vi "TestTriggerTimestamp.vi"() -> ()   [LabVIEW 2014]
uses:
  <instrlib>/niSync/niSync.llb/niSync Initialize (IVI).vi
  <instrlib>/niSync/niSync.llb/niSync Set Time Reference (GPS).vi
  <instrlib>/niSync/niSync.llb/niSync Create Clock (Frequency).vi
  <instrlib>/niSync/niSync.llb/niSync Read Trigger Time Stamp (Single).vi
panel:
  out "Final error":errorcluster
  out "Connection Error":errorcluster
  in  "source terminal":string(combo)="PXI_Trig2"
  out "Stop":bool
  out "Pause Error":errorcluster
  out "Play Error":errorcluster
  in  "Trigger Terminal":tag="/PXI1Slot7/PFI1"
  in  "Reference Clock":refnum<k15>="PXI1Slot7"
  out "time stamp out":timestamp
  out "Read Error":errorcluster
  in  "Pause Button":bool
  in  "Play Button":bool
  in  "Stop Button":bool
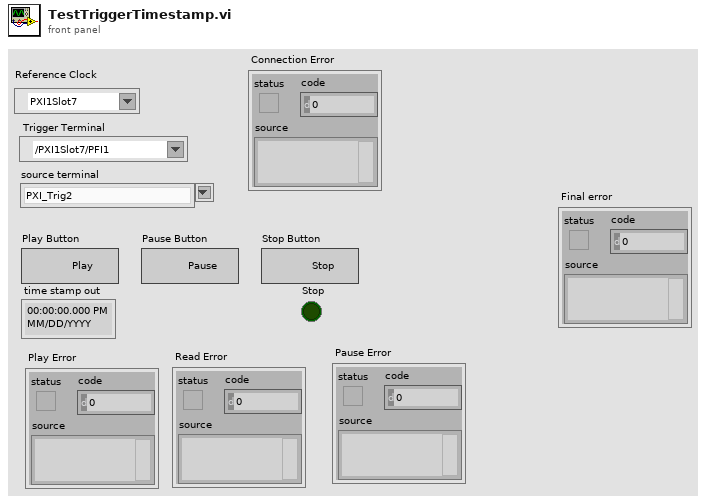
[diagram p1: front panel]
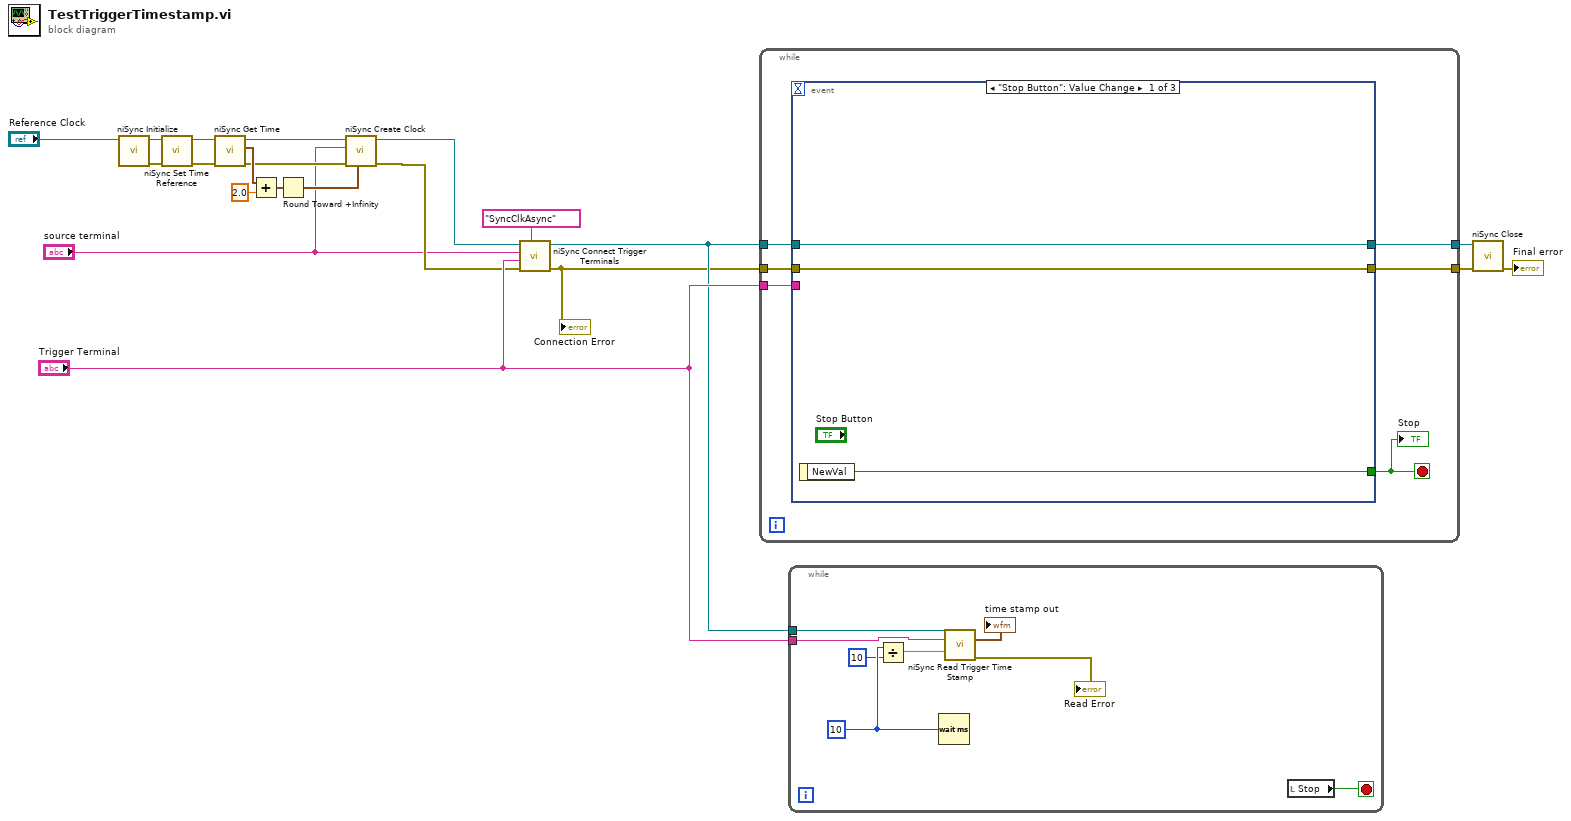
[diagram p0: block diagram]
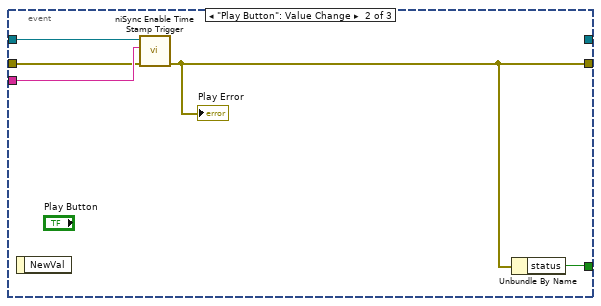
[diagram p2: hidden frame]
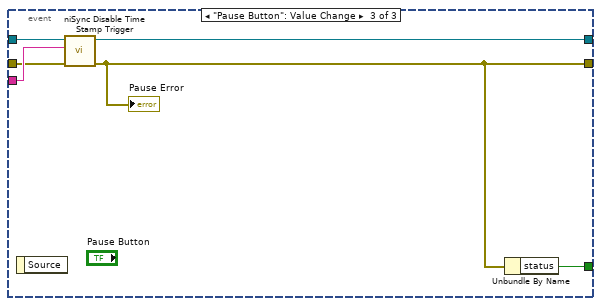
[diagram p3: hidden frame]
diagram:
  n1 = call-poly <instrlib>:"niSync Initialize.vi"("resource name"="Reference Clock") -> ("error out"=w19:errorcluster, "instrument handle out"=w20:refnum<k15>)  [unwired: 9 in]
  n2 = call-poly <instrlib>:"niSync Set Time Reference.vi"("error in (no error)"=w19, "instrument handle"=w20) -> ("error out"=w17:errorcluster, "instrument handle out"=w18:refnum<k15>)  [unwired: 8 in]
  n3 = call <instrlib>:"niSync Get Time.vi"("error in (no error)"=w17, "instrument handle"=w18) -> ("error out"=w11:errorcluster, "time"=w15:timestamp, "instrument handle out"=w16:refnum<k15>)  [unwired: 5 in]
  n4 = Add(x=w15, y=2.0) -> (x+y=w13:timestamp)
  n5 = Round Toward +Infinity(x=w13) -> (ceil(x): smallest int >= x=w12:timestamp)
  n6 = call-poly <instrlib>:"niSync Create Clock.vi"("start time"=w12, "error in (no error)"=w11, "terminal"="source terminal", "instrument handle"=w16) -> ("error out"=w9:errorcluster, "instrument handle out"=w8:refnum<k15>)  [unwired: 4 in, 2 out]
  n7 = call <instrlib>:"niSync Connect Trigger Terminals.vi"("synchronization clock"="SyncClkAsync", "error in (no error)"=w9, "destination terminal"="Trigger Terminal", "source terminal"="source terminal", "instrument handle"=w8) -> ("error out"=w1:errorcluster, "instrument handle out"=w2:refnum<k15>)  [unwired: 5 in]
  "Connection Error" <- w1
  n8 = while {
    tunnel: w2 -> [w27]
    tunnel: "Trigger Terminal" -> [w26]
    tunnel: [w25] -> w7
    tunnel: [w24] -> w6
    tunnel: w1 -> [w23]
    stop <- w22 stop-if-true
    n9 = event shown="[0] \"Stop Button\": Value Change" {
      selector: _ -> [_ _ _]
      dyn-events: _ -> [_ _ _]
      timeout: _ -> [_ _ _]
      tunnel: [w28 w31 w36] -> w22
      tunnel: w27 -> [w30 w35 w41]
      tunnel: w26 -> [_ w34 w40]
      tunnel: [w30 _ w37] -> w25
      tunnel: [w29 w32 w38] -> w24
      tunnel: w23 -> [w29 w33 w39]
      event "Stop Button": Value Change {
        n10 = event-data() -> ("NewVal"=w28:bool)  [unwired: 1 in]
      }
      event "Play Button": Value Change {
        n11 = event-data() -> ()  [unwired: 1 in, 1 out]
        n12 = call <instrlib>:"niSync Enable Time Stamp Trigger.vi"("error in (no error)"=w33, "terminal"=w34, "instrument handle"=w35) -> ("error out"=w32:errorcluster)  [unwired: 6 in, 1 out]
        "Play Error" <- w32
        n13 = Unbundle By Name(w32) -> ("status"=w31:bool)
      }
      event "Pause Button": Value Change {
        n14 = event-data() -> ()  [unwired: 1 in, 1 out]
        n15 = call <instrlib>:"niSync Disable Time Stamp Trigger.vi"("error in (no error)"=w39, "terminal"=w40, "instrument handle"=w41) -> ("error out"=w38:errorcluster, "instrument handle out"=w37:refnum<k15>)  [unwired: 6 in]
        "Pause Error" <- w38
        n16 = Unbundle By Name(w38) -> ("status"=w36:bool)
      }
    }
    "Stop" <- w22
  }
  n17 = while {
    tunnel: w2 -> [w44]
    tunnel: "Trigger Terminal" -> [w43]
    stop <- w42 stop-if-true
    w48 = u32 10 ("milliseconds to wait")
    n18 = Divide(x=w48, y=u32 10) -> (x/y=w49:dbl)
    n19 = Wait (ms)(milliseconds to wait=w48) -> ()  [unwired: 1 out]
    n20 = call-poly <instrlib>:"niSync Read Trigger Time Stamp.vi"("instrument handle"=w44, "terminal"=w43, "timeout"=w49) -> ("time stamp out"=→"time stamp out":timestamp, "error out"=→"Read Error":errorcluster)  [unwired: 9 in, 2 out]
    n21 = local read "Stop"() -> (w42:bool)
  }
  n22 = call <instrlib>:"niSync Close.vi"("error in (no error)"=w6, "instrument handle"=w7) -> ("error out"=→"Final error":errorcluster)  [unwired: 9 in]
